vi "Teleop.vi"(10 "Match Info":T1={"Autonomous Elapsed Seconds"=0.0, "TeleOp Elapsed Seconds"=0.0, "Disabled Elapsed Seconds"=0.0, "Visited Autonomous"=FALSE, "Visited TeleOp"=FALSE, "Visited Disabled"=FALSE, "Autonomous Settings"={"Autonomous Style"=enum."Independent", "VI Refnum"=refnum}}, 11 "Call Context":T2) -> ()   [LabVIEW 2013]
doc: "This VI is called for each TeleOp packet received from the DS where the robot is not disabled. It is often used to read from the joysticks and update I/O or to update setpoints for timed control loops. It should complete and return within 20 milliseconds or it may miss DS packets."
uses:
  <vilib>/Rock Robotics/WPI/DriverStation/WPI_DriverStationDerivedRobotMode.ctl
  <vilib>/Rock Robotics/WPI/DriverStation/WPI_DriverStationMatch Info.ctl
  Robot Global Data.vi
  <vilib>/Rock Robotics/WPI/Joystick/WPI_JoystickGetSetRefNum.vi
panel:
  in  "HarvSpeed":dbl=0.5
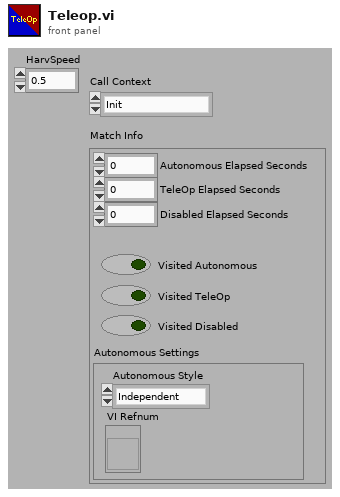
[diagram p1: front panel]
types:
  T1 = typedef "WPI_DriverStationMatch Info.ctl" = cluster{"Autonomous Elapsed Seconds":dbl, "TeleOp Elapsed Seconds":dbl, "Disabled Elapsed Seconds":dbl, "Visited Autonomous":bool, "Visited TeleOp":bool, "Visited Disabled":bool, "Autonomous Settings":cluster{"Autonomous Style":enum16{"Iterative", "Independent"}, "VI Refnum":refnum<vi>}}
  T2 = typedef "WPI_DriverStationDerivedRobotMode.ctl" = enum16{"Init", "Execute", "Stop"}
  T3 = typedef "WPI_JoystickDevRef.ctl" = cluster{"Device":T4}
  T4 = typedef "WPI_JoystickDeviceEnum.ctl" = enum16{"USB 1", "USB 2", "USB 3", "USB 4", "Kinect 1", "Kinect 2"}
  T5 = cluster{"axis 1 (x)":dbl, "axis 2 (y)":dbl, "axis 3 (throttle)":dbl, "axis 4":dbl, "axis 5":dbl, "axis 6":dbl}
  T6 = typedef "WPI_MotorControlDeviceRef.ctl" = cluster{"DeviceStatus":errorcluster, "Type":enum16{"PWM", "CAN"}, "PWM":cluster{"Digital Module":T7, "PWM Channel":T8, "DeadBand":T9}, "CAN":cluster{"Device Number":u8, "Control Mode":T10, "Semaphore":T11, "Max Vout":dbl}, "Invert":bool, "TransformRef":T12, "InvTransformRef":T12}
  T7 = typedef "FPGA_TypedefDigitalModule.ctl" = enum16{"Digital Module 1", "Digital Module 2"}
  T8 = typedef "FPGA_DIOPWMChannel.ctl" = enum8{"PWM 1", "PWM 2", "PWM 3", "PWM 4", "PWM 5", "PWM 6", "PWM 7", "PWM 8", "PWM 9", "PWM 10", "Invalid"}
  T9 = typedef "WPI_PWMDeadband.ctl" = cluster{"Name":string, "maxPositivePwm":i32, "minPositivePwm":i32, "centerPwm":i32, "maxNegativePwm":i32, "minNegativePwm":i32, "angularRange":u16}
  T10 = typedef "WPI_CANJaguar_ControlMode.ctl" = enum8{"Percent VBus", "Current", "Speed", "Position", "Voltage"}
  T11 = typedef "Semaphore RefNum" = refnum<k1>
  T12 = typedef "WPI_PWMTransform_ConPane.ctl" = refnum<vi>
  T13 = cluster{"Driver Station Digital Input (1-8)[0]":bool, "Driver Station Digital Input (1-8)[1]":bool, "Driver Station Digital Input (1-8)[2]":bool, "Driver Station Digital Input (1-8)[3]":bool, "Driver Station Digital Input (1-8)[4]":bool, "Driver Station Digital Input (1-8)[5]":bool, "Driver Station Digital Input (1-8)[6]":bool, "Driver Station Digital Input (1-8)[7]":bool, "Driver Station Digital Input (1-8)[8]":bool}
  T14 = cluster{"RightLow":dbl, "LeftLow":dbl, "RightHigh":dbl, "LeftHigh":dbl}
  T15 = typedef "WPI_JoystickButtonState.ctl" = cluster{"Button 1":bool, "Button 2":bool, "Button 3":bool, "Button 4":bool, "Button 5":bool, "Button 6":bool, "Button 7":bool, "Button 8":bool, "Button 9":bool, "Button 10":bool, "Button 11":bool, "Button 12":bool}
  T16 = typedef "WPI_ServoDeviceRef.ctl" = cluster{"DeviceStatus":errorcluster, "Digital Module":T7, "PWM Channel":T8, "DeadBand":T9}
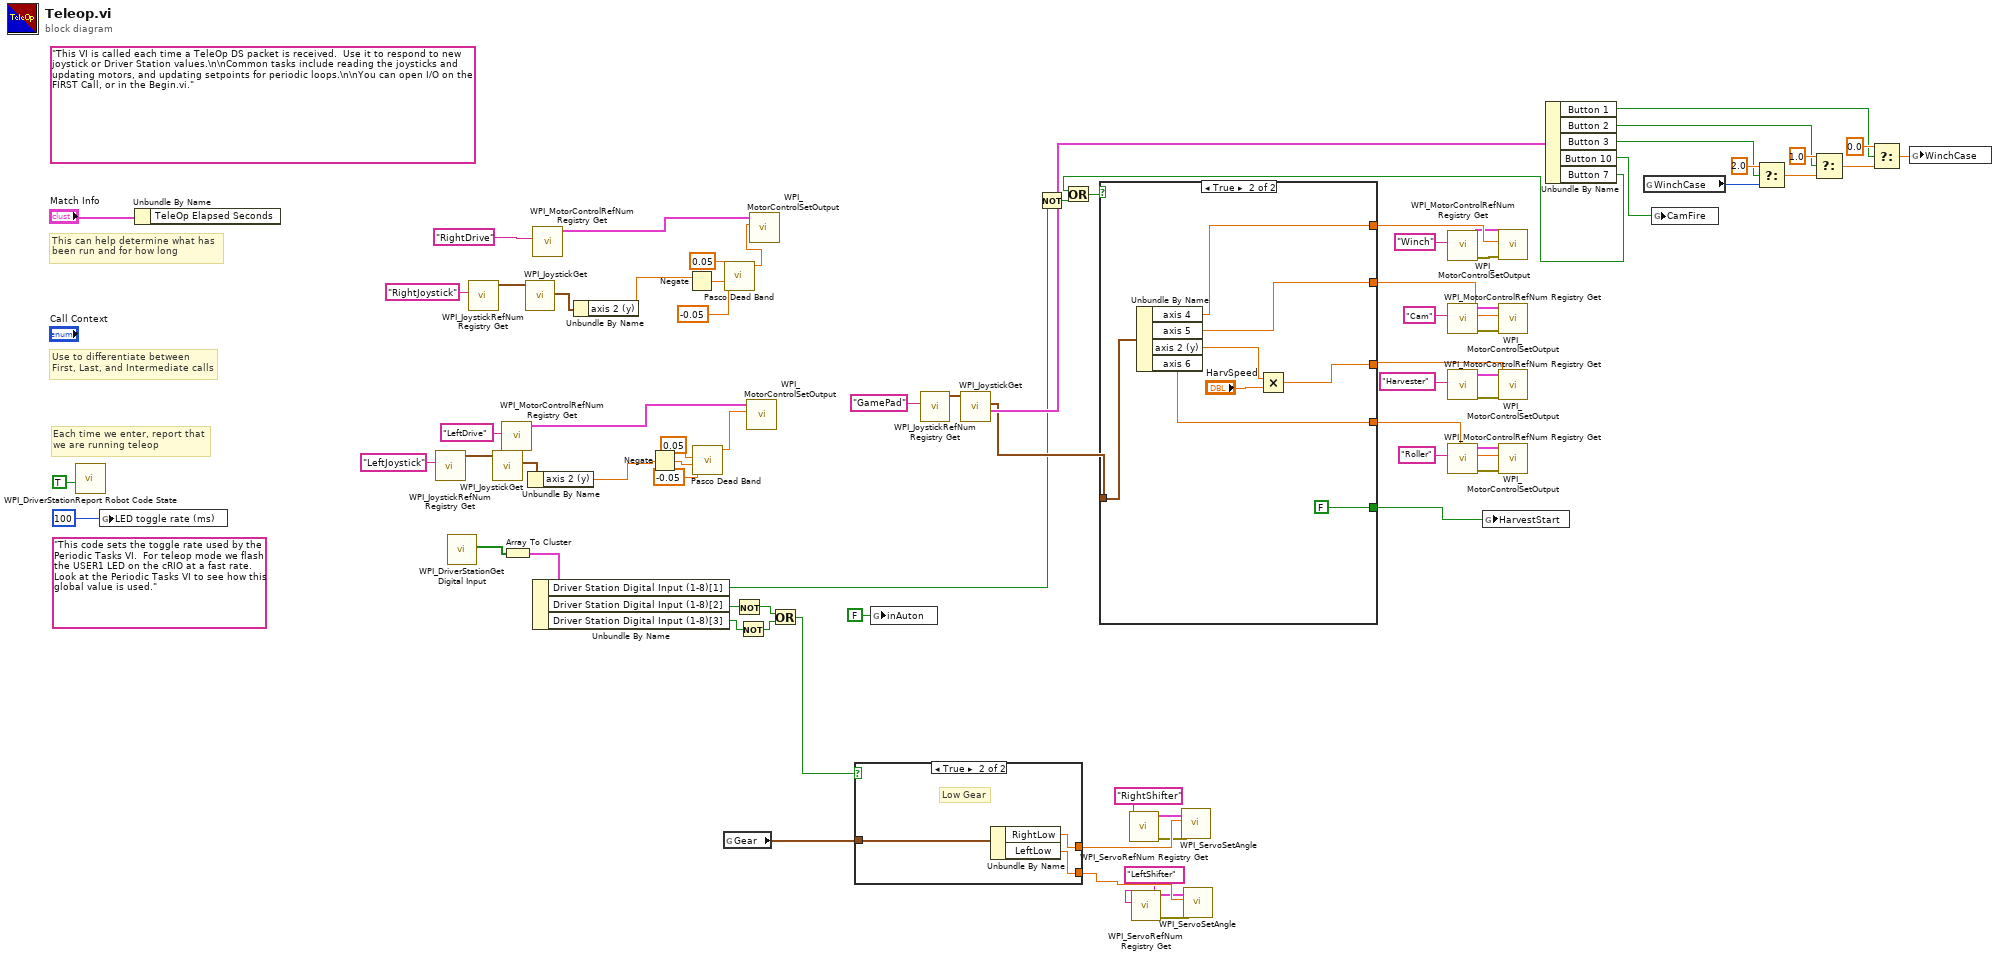
[diagram p0: block diagram]
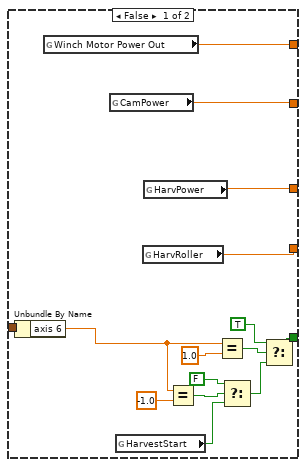
[diagram p2: hidden frame]
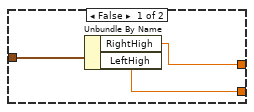
[diagram p3: hidden frame]
diagram:
  (unwired) "This code sets the toggle rate used by the Periodic Tasks VI.  For teleop mode we flash the USER1 LED on the cRIO at a fast rate.  Look at the Periodic Tasks VI to see how this global value is used."
  (unwired) "This VI is called each time a TeleOp DS packet is received.  Use it to respond to new joystick or Driver Station values.\n\nCommon tasks include reading the joysticks and updating motors, and updating setpoints for periodic loops.\n\nYou can open I/O on the FIRST Call, or in the Begin.vi."
  # "Each time we enter, report that\nwe are running teleop"
  # "Use to differentiate between\nFirst, Last, and Intermediate calls"
  # "This can help determine what has\nbeen run and for how long"
  n1 = call <vilib>:"WPI_DriverStationReport Robot Code State.vi"("TeleOp"=TRUE ("Autonomous")) -> ()  [unwired: 10 in, 1 out]
  n2 = global write "Robot Global Data.vi" "LED toggle rate (ms)"(u32 100 ("LED ms toggle rate")) -> ()
  n3 = Unbundle By Name("Match Info") -> ()  [unwired: 1 out]
  n4 = call <vilib>:"WPI_JoystickRefNum Registry Get.vi"("refnum name"="LeftJoystick") -> ("JoystickDevRef"=w65:T3)  [unwired: 9 in, 1 out]
  n5 = call <vilib>:"WPI_DriverStationGet Digital Input.vi"() -> ("Driver Station Digital Input (1-8)"=w16:bool[])  [unwired: 11 in]
  n6 = call <vilib>:"WPI_JoystickRefNum Registry Get.vi"("refnum name"="RightJoystick") -> ("JoystickDevRef"=w70:T3)  [unwired: 9 in, 1 out]
  n7 = call <vilib>:"WPI_JoystickGet.vi"("JoystickDevRef"=w65) -> ("Axes"=w64:T5)  [unwired: 4 in, 2 out]
  n8 = call <vilib>:"WPI_MotorControlRefNum Registry Get.vi"("refnum name"="LeftDrive") -> ("MotorControlDevRef"=w68:T6)  [unwired: 9 in, 1 out]
  n9 = Array To Cluster(array=w16) -> (cluster=w15:T13)
  n10 = call <vilib>:"WPI_JoystickGet.vi"("JoystickDevRef"=w70) -> ("Axes"=w69:T5)  [unwired: 4 in, 2 out]
  n11 = Unbundle By Name(w64) -> ("axis 2 (y)"=w63:dbl)
  n12 = call <vilib>:"WPI_MotorControlRefNum Registry Get.vi"("refnum name"="RightDrive") -> ("MotorControlDevRef"=w73:T6)  [unwired: 9 in, 1 out]
  n13 = Unbundle By Name(w15) -> ("Driver Station Digital Input (1-8)[1]"=w14:bool, "Driver Station Digital Input (1-8)[2]"=w5:bool, "Driver Station Digital Input (1-8)[3]"=w4:bool)
  n14 = Unbundle By Name(w69) -> ("axis 2 (y)"=w62:dbl)
  n15 = Negate(x=w63) -> (-x=w57:dbl)
  n16 = Negate(x=w62) -> (-x=w61:dbl)
  n17 = call "Pasco Dead Band.vi"("lower limit"=-0.05, "PWM Power"=w57, "upper limit"=0.05) -> ("PWM Power"=w54:dbl)  [unwired: 7 in, 1 out]
  n18 = global read "Robot Global Data.vi" "Gear"() -> (w53:T14)
  n19 = call "Pasco Dead Band.vi"("lower limit"=-0.05, "PWM Power"=w61, "upper limit"=0.05) -> ("PWM Power"=w60:dbl)  [unwired: 7 in, 1 out]
  n20 = Not(x=w5) -> (.not. x?=w2:bool)
  n21 = Not(x=w4) -> (.not. x?=w3:bool)
  n22 = call <vilib>:"WPI_MotorControlSetOutput.vi"("Output"=w54, "MotorControlDevRef"=w68) -> ()  [unwired: 7 in, 3 out]
  n23 = call <vilib>:"WPI_MotorControlSetOutput.vi"("Output"=w60, "MotorControlDevRef"=w73) -> ()  [unwired: 7 in, 3 out]
  n24 = Or(x=w2, y=w3) -> (x .or. y?=w1:bool)
  n25 = case shown="True" w1 {
    tunnel: w53 -> [w79 w82]
    tunnel: [w78 w81] -> w52
    tunnel: [w77 w80] -> w51
    frame False {
      n26 = Unbundle By Name(w79) -> ("RightHigh"=w78:dbl, "LeftHigh"=w77:dbl)
    }
    frame True {
      # "Low Gear"
      n27 = Unbundle By Name(w82) -> ("RightLow"=w81:dbl, "LeftLow"=w80:dbl)
    }
  }
  n28 = global write "Robot Global Data.vi" "inAuton"(FALSE ("inAuton")) -> ()
  n29 = call <vilib>:"WPI_JoystickRefNum Registry Get.vi"("refnum name"="GamePad") -> ("JoystickDevRef"=w49:T3)  [unwired: 9 in, 1 out]
  n30 = call <vilib>:"WPI_JoystickGet.vi"("JoystickDevRef"=w49) -> ("Buttons"=w22:T15, "Axes"=w20:T5)  [unwired: 4 in, 1 out]
  n31 = Not(x=w14) -> (.not. x?=w13:bool)
  n32 = call <vilib>:"WPI_ServoRefNum Registry Get.vi"("refnum name"="RightShifter") -> ("error out"=w11:errorcluster, "ServoDeviceRef"=w10:T16)  [unwired: 9 in]
  n33 = call <vilib>:"WPI_ServoRefNum Registry Get.vi"("refnum name"="LeftShifter") -> ("error out"=w7:errorcluster, "ServoDeviceRef"=w8:T16)  [unwired: 9 in]
  n34 = call <vilib>:"WPI_ServoSetAngle.vi"("error in (no error)"=w11, "Angle"=w52, "ServoDeviceRef"=w10) -> ()  [unwired: 7 in, 2 out]
  n35 = call <vilib>:"WPI_ServoSetAngle.vi"("error in (no error)"=w7, "Angle"=w51, "ServoDeviceRef"=w8) -> ()  [unwired: 7 in, 2 out]
  n36 = call <vilib>:"WPI_MotorControlRefNum Registry Get.vi"("refnum name"="Winch") -> ("error out"=w40:errorcluster, "MotorControlDevRef"=w34:T6)  [unwired: 9 in]
  n37 = call <vilib>:"WPI_MotorControlRefNum Registry Get.vi"("refnum name"="Cam") -> ("error out"=w39:errorcluster, "MotorControlDevRef"=w38:T6)  [unwired: 9 in]
  n38 = call <vilib>:"WPI_MotorControlRefNum Registry Get.vi"("refnum name"="Harvester") -> ("error out"=w44:errorcluster, "MotorControlDevRef"=w43:T6)  [unwired: 9 in]
  n39 = call <vilib>:"WPI_MotorControlRefNum Registry Get.vi"("refnum name"="Roller") -> ("error out"=w46:errorcluster, "MotorControlDevRef"=w47:T6)  [unwired: 9 in]
  n40 = Unbundle By Name(w22) -> ("Button 1"=w25:bool, "Button 2"=w26:bool, "Button 3"=w27:bool, "Button 10"=w21:bool, "Button 7"=w17:bool)
  n41 = Or(x=w17, y=w13) -> (x .or. y?=w18:bool)
  n42 = case shown="True" w18 {
    tunnel: [w97 w104] -> w45
    tunnel: [w96 w99] -> w41
    tunnel: w20 -> [w84 w105]
    tunnel: [w94 w103] -> w35
    tunnel: [w95 w102] -> w33
    tunnel: [w83 FALSE ("HarvestStart")] -> w19
    frame False {
      n43 = Unbundle By Name(w84) -> ("axis 6"=w92:dbl)
      n44 = global read "Robot Global Data.vi" "Winch Motor Power Out"() -> (w94:dbl)
      n45 = global read "Robot Global Data.vi" "CamPower"() -> (w95:dbl)
      n46 = global read "Robot Global Data.vi" "HarvestStart"() -> (w93:bool)
      n47 = global read "Robot Global Data.vi" "HarvRoller"() -> (w97:dbl)
      n48 = global read "Robot Global Data.vi" "HarvPower"() -> (w96:dbl)
      n49 = Equal?(x=w92, y=-1.0) -> (x = y?=w91:bool)
      n50 = Equal?(x=w92, y=1.0) -> (x = y?=w86:bool)
      n51 = Select(t=FALSE, s=w91, f=w93) -> (s? t:f=w89:bool)
      n52 = Select(t=TRUE, s=w86, f=w89) -> (s? t:f=w83:bool)
    }
    frame True {
      n53 = Unbundle By Name(w105) -> ("axis 4"=w103:dbl, "axis 5"=w102:dbl, "axis 2 (y)"=w100:dbl, "axis 6"=w104:dbl)
      n54 = Multiply(x=w100, y="HarvSpeed") -> (x*y=w99:dbl)
    }
  }
  n55 = global write "Robot Global Data.vi" "HarvestStart"(w19) -> ()
  n56 = call <vilib>:"WPI_MotorControlSetOutput.vi"("error in (no error)"=w40, "Output"=w35, "MotorControlDevRef"=w34) -> ()  [unwired: 6 in, 3 out]
  n57 = call <vilib>:"WPI_MotorControlSetOutput.vi"("error in (no error)"=w39, "Output"=w33, "MotorControlDevRef"=w38) -> ()  [unwired: 6 in, 3 out]
  n58 = call <vilib>:"WPI_MotorControlSetOutput.vi"("error in (no error)"=w44, "Output"=w41, "MotorControlDevRef"=w43) -> ()  [unwired: 6 in, 3 out]
  n59 = call <vilib>:"WPI_MotorControlSetOutput.vi"("error in (no error)"=w46, "Output"=w45, "MotorControlDevRef"=w47) -> ()  [unwired: 6 in, 3 out]
  n60 = global read "Robot Global Data.vi" "WinchCase"() -> (w23:i32)
  n61 = global write "Robot Global Data.vi" "CamFire"(w21) -> ()
  n62 = Select(t=2.0, s=w27, f=w23) -> (s? t:f=w32:dbl)
  n63 = Select(t=1.0, s=w26, f=w32) -> (s? t:f=w31:dbl)
  n64 = Select(t=0.0, s=w25, f=w31) -> (s? t:f=w24:dbl)
  n65 = global write "Robot Global Data.vi" "WinchCase"(w24) -> ()
